vi "OAT Tachless Add Del Order List.vi"(9 "Order":dbl format="%.2f", 10 "List Ctl":cluster{"Add":bool, "Del":bool}, 11 "Order List ref":refnum<vi>) -> ()   [LabVIEW 2017, in "SoundVib_Tachless.lvlib"]
uses:
  <vilib>/addons/Sound and Vibration/Order Analysis/Tachless/SoundVib_Tachless.lvlib
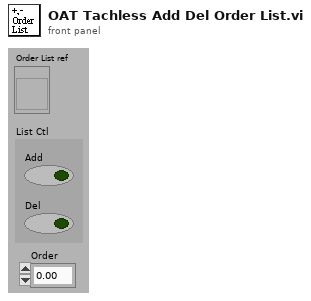
[diagram p1: front panel]
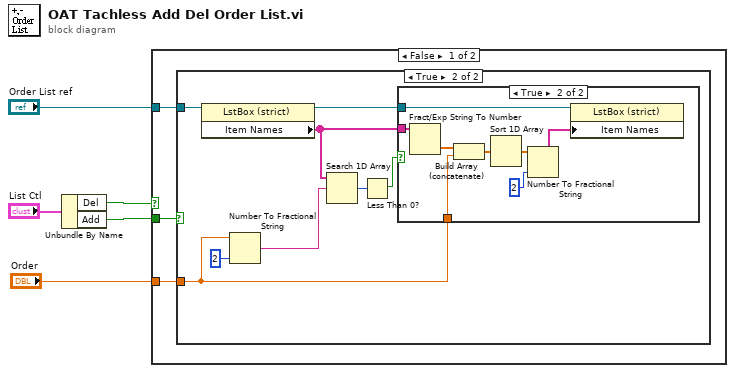
[diagram p0: block diagram]
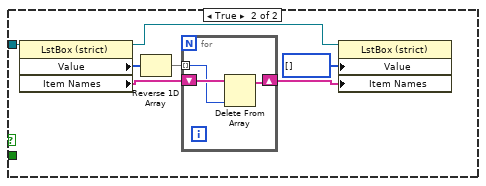
[diagram p4: hidden frame]
diagram:
  n1 = Unbundle By Name("List Ctl") -> ("Del"=w4:bool, "Add"=w1:bool)
  n2 = case shown="False" w4 {
    tunnel: "Order List ref" -> [w8 w28]
    tunnel: "Order" -> [w7 _]
    tunnel: w1 -> [w6 _]
    frame False {
      n3 = case shown="True" w6 {
        tunnel: w8 -> [_ w16]
        tunnel: w7 -> [_ w14]
        frame False {
        }
        frame True {
          n4 = property on="Property Node" class="LstBox (strict)"(reference=w16) -> (reference out=w15:refnum<vi>, "Item Names"=w12:string[])  [unwired: 1 in, 1 out]
          n5 = Number To Fractional String(number=w14, precision (6)=i16 2) -> (F-format string=w11:string)  [unwired: 2 in]
          n6 = Search 1D Array(1D array=w12, element=w11) -> (index of element=w10:i32)  [unwired: 1 in]
          n7 = Less Than 0?(x=w10) -> (x < 0?=w9:bool)
          n8 = case shown="True" w9 {
            tunnel: w15 -> [_ w21]
            tunnel: w14 -> [_ w18]
            tunnel: w12 -> [_ w17]
            frame False {
            }
            frame True {
              n9 = Fract/Exp String To Number(string=w17) -> (number=w23:dbl[])  [unwired: 3 in, 1 out]
              n10 = Build Array (concatenate)(w23, w18) -> (w22:dbl[])
              n11 = Sort 1D Array(array=w22) -> (sorted array=w19:dbl[])
              n12 = Number To Fractional String(number=w19, precision (6)=i16 2) -> (F-format string=w20:string[])  [unwired: 2 in]
              n13 = property on="Property Node" class="LstBox (strict)"(reference=w21, "Item Names"=w20) -> ()  [unwired: 1 in, 2 out]
            }
          }
        }
      }
    }
    frame True {
      n14 = property on="Property Node" class="LstBox (strict)"(reference=w28) -> (reference out=w25:refnum<vi>, "Value"=w31:i32[], "Item Names"=w30:string[])  [unwired: 1 in, 1 out]
      n15 = Reverse 1D Array(array=w31) -> (reversed array=w29:i32[])
      n16 = for {
        shift-right: [w32] -> w27
        shift-left: w30 -> [w34]
        tunnel: w29 -> [w33] mode=indexing
        n17 = Delete From Array(array=w34, index=w33) -> (array with subset deleted=w32:string[])  [unwired: 1 in, 1 out]
      }
      n18 = property on="Property Node" class="LstBox (strict)"(reference=w25, "Value"=i32[] [], "Item Names"=w27) -> ()  [unwired: 1 in, 2 out]
    }
  }
